vi "Request Callback VI Type.vi"(7 "Owner":refnum<class>, 9 "URI Params":string[](array[string]), 10 "Request":refnum<class "Request.lvclass">, 11 "Server":refnum<class "Server.lvclass">) -> (0 "error out":errorcluster, 2 "Response":refnum<class "Response.lvclass">)   [LabVIEW 2020, in "HTTP Server.lvlib"]
uses:
  HTTP Server.lvlib
  Server/Server.lvclass
  <vilib>/IlluminatedG/IG HTTP Utils/HTTP Utils/Request/Request.lvclass
  <vilib>/IlluminatedG/IG HTTP Utils/HTTP Utils/Response/Response.lvclass
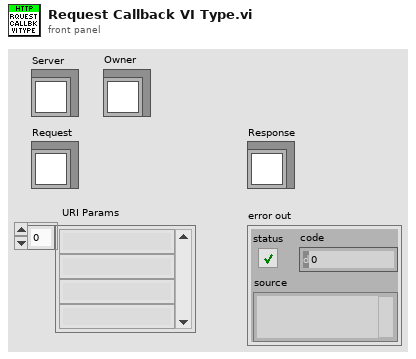
[diagram p1: front panel]
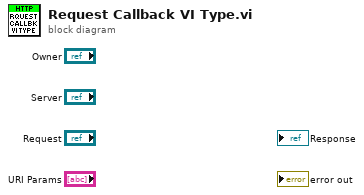
[diagram p0: block diagram]
diagram:
